vi "Extrapolate.vi"(9 "Polynomial Coefficients":dbl[](array[numeric]), 10 "xi":dbl[](array[numeric])) -> (2 "yi":dbl[](array[numeric]))   [LabVIEW 2009]
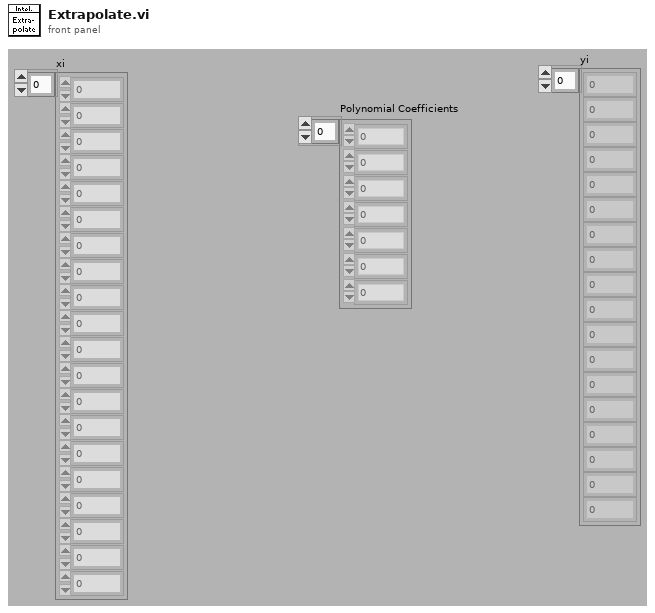
[diagram p1: front panel]
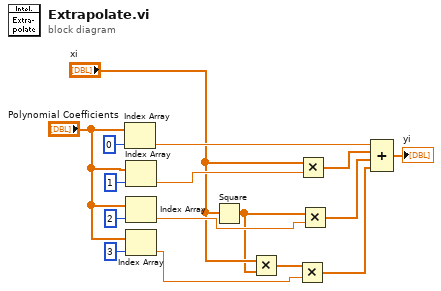
[diagram p0: block diagram]
diagram:
  n1 = Index Array(array="Polynomial Coefficients", index=0) -> (element=w9:dbl)
  n2 = Index Array(array="Polynomial Coefficients", index=1) -> (element=w11:dbl)
  n3 = Index Array(array="Polynomial Coefficients", index=2) -> (element=w10:dbl)
  n4 = Index Array(array="Polynomial Coefficients", index=3) -> (element=w1:dbl)
  n5 = Square(x="xi") -> (x^2=w5:dbl[])
  n6 = Multiply(x="xi", y=w5) -> (x*y=w3:dbl[])
  n7 = Multiply(x=w3, y=w1) -> (x*y=w2:dbl[])
  n8 = Multiply(x="xi", y=w11) -> (x*y=w8:dbl[])
  n9 = Multiply(x=w5, y=w10) -> (x*y=w7:dbl[])
  n10 = Compound Arithmetic op=ADD(w9, w8, w7, w2) -> (→"yi":dbl[])
